vi "DRV_SDSU_set_gain_and_speed.vi"(0 "fd":i32, 5 "gain":i32, 7 "speed":i32, 11 "error in (no error)":errorcluster) -> (4 "fd out":i32, 8 "return value":i32, 15 "error out":errorcluster)   [LabVIEW 2016]
doc: "This VI closes the I/O interface with the instrument."
uses:
  c/lib/libarcDHE.so
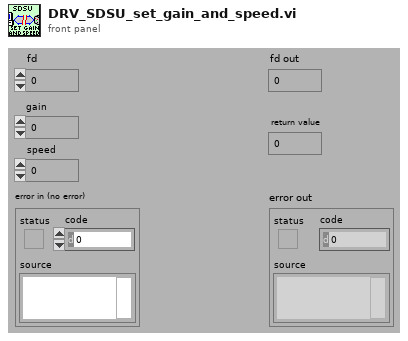
[diagram p1: front panel]
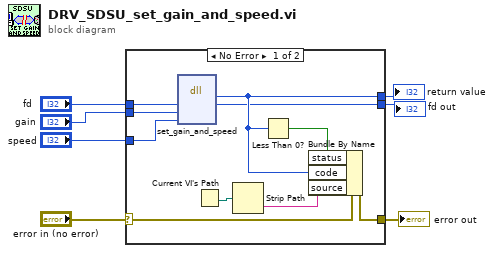
[diagram p0: block diagram]
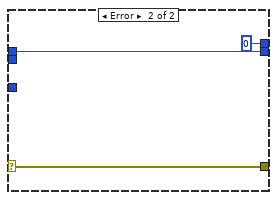
[diagram p2: hidden frame]
diagram:
  n1 = case shown="No Error" "error in (no error)" {
    selector: "error in (no error)" -> [w8 w18]
    tunnel: "fd" -> [w17 w20]
    tunnel: [w15 0] -> w6
    tunnel: [w12 w18] -> w5
    tunnel: "gain" -> [w11 _]
    tunnel: "speed" -> [w10 _]
    tunnel: [w9 w20] -> w2
    frame No Error {
      n2 = dll-call lib="home/sensei/panview/PAN/Modules/SDSU/private/c/lib/libarcDHE.so" fn="set_gain_and_speed"("fd"=w17, "gain"=w11, "speed"=w10) -> ("return type"=w15:i32, "fd"=w9:i32)  [unwired: 5 in, 2 out]
      n3 = Current VI's Path() -> (path=w14:path)
      n4 = Strip Path(path=w14) -> (name=w13:string)  [unwired: 1 out]
      n5 = Less Than 0?(x=w15) -> (x < 0?=w16:bool)
      n6 = Bundle By Name(cluster=w8, "status"=w16, "code"=w15, "source"=w13) -> (w12:errorcluster)
    }
    frame Error {
    }
  }
  "error out" <- w5
  "return value" <- w6
  "fd out" <- w2
